vi "process.vi"(8 "error in (no error)":errorcluster, 11 "Library in":refnum<class "Library.lvclass">) -> (0 "error out":errorcluster, 3 "Library out":refnum<class "Library.lvclass">)   [LabVIEW 2016, in "Library.lvclass"]
uses:
  Library.lvclass
  C:/LSST_TS/SystemSW/ct_tools/ProjectItem/ProjectItem.lvclass
  ProjectItem/ProjectItem.lvclass/ProjectItem.ctl
  Search/Search.lvclass/Search.ctl
  IProjectItemFactory/IProjectItemFactory.lvclass
  ProjectItem/ProjectItem.lvclass
  Project/Project.lvclass
  Search/Search.lvclass
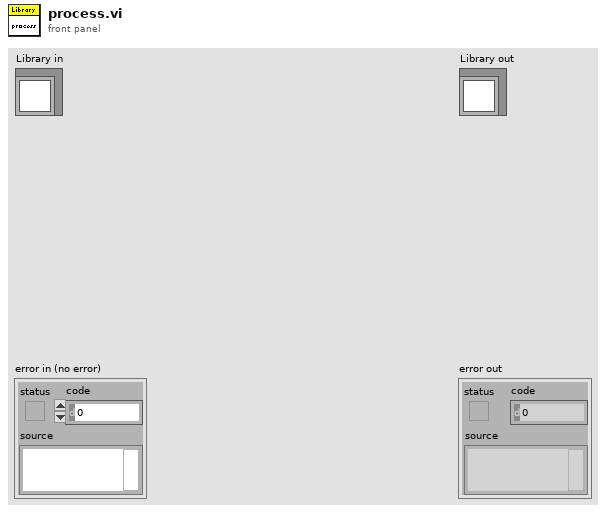
[diagram p1: front panel]
types:
  T1 = typedef "ProjectItemSelection.ctl" = enum16{"Default", "ClassPrivateData", "Dependencies", "Folder", "Library", "LVClass", "VI"}
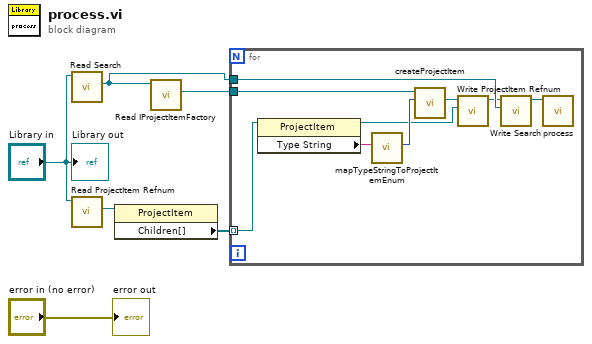
[diagram p0: block diagram]
diagram:
  n1 = call "Read Search.vi"("ProjectItem in"="Library in") -> ("Search"=w1:refnum<class "Search.lvclass">)  [unwired: 9 in, 1 out]
  n2 = call "Read ProjectItem Refnum.vi"("ProjectItem in"="Library in") -> ("ProjectItem Refnum"=w5:refnum<vi>)  [unwired: 9 in, 1 out]
  n3 = property class="ProjectItem"(reference=w5) -> ("Children[]"=w4:refnum<vi>[])  [unwired: 1 in, 2 out]
  n4 = call "Read IProjectItemFactory.vi"("ProjectItem in"=w1) -> ("IProjectItemFactory"=w2:refnum<class "IProjectItemFactory.lvclass">)  [unwired: 9 in, 1 out]
  n5 = for {
    tunnel: w4 -> [w15] mode=indexing
    tunnel: w2 -> [w11]
    tunnel: w1 -> [w9]
    n6 = property class="ProjectItem"(reference=w15) -> (reference out=w10:refnum<vi>, "Type String"=w14:string)  [unwired: 1 in, 1 out]
    n7 = call "mapTypeStringToProjectItemEnum.vi"("Type String"=w14) -> ("ProjectItemSelection"=w13:T1)  [unwired: 8 in, 2 out]
    n8 = call-dynamic "createProjectItem.vi"("ProjectItemSelection"=w13, "IProjectItemFactory in"=w11) -> ("ProjectItem"=w12:refnum<class "ProjectItem.lvclass">)  [unwired: 7 in, 2 out]
    n9 = call "Write ProjectItem Refnum.vi"("ProjectItem Refnum"=w10, "ProjectItem in"=w12) -> ("ProjectItem out"=w8:refnum<class "ProjectItem.lvclass">)  [unwired: 9 in]
    n10 = call "Write Search.vi"("Search"=w9, "ProjectItem in"=w8) -> ("ProjectItem out"=w7:refnum<class "ProjectItem.lvclass">)  [unwired: 9 in]
    n11 = call-dynamic "process.vi"("ProjectItem in"=w7) -> ()  [unwired: 9 in, 2 out]
  }
  "error out" <- "error in (no error)"
  "Library out" <- "Library in"
